vi "PrvwShift.vi"(8 "Preview Shift":i32, 11 "Input Array":dbl[](array[numeric])) -> (3 "Output Array":dbl[](array[numeric]))   [LabVIEW 2016]
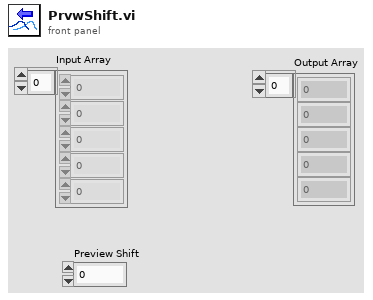
[diagram p1: front panel]
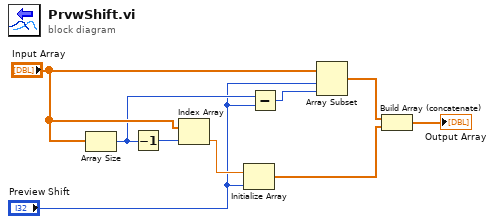
[diagram p0: block diagram]
diagram:
  n1 = Array Size(array="Input Array") -> (size(s)=w5:i32)
  n2 = Decrement(x=w5) -> (x-1=w9:i32)
  n3 = Index Array(array="Input Array", index=w9) -> (element=w8:dbl)
  n4 = Initialize Array(w8, "Preview Shift") -> (w3:dbl[])
  n5 = Subtract(x=w5, y="Preview Shift") -> (x-y=w6:i32)
  n6 = Array Subset(array="Input Array", index="Preview Shift", length=w6) -> (w2:dbl[])
  n7 = Build Array (concatenate)(w2, w3) -> (→"Output Array":dbl[])
